vi "Configure Dialog.vi"(8 "error in (no error)":errorcluster, 11 "Create Channel Arbitrary Waveform [ACH] Msg in":refnum<class "Create Channel Arbitrary Waveform [ACH] Msg.lvclass">) -> (0 "error out":errorcluster, 2 "Ok?":bool, 3 "Create Channel Arbitrary Waveform [ACH] Msg out":refnum<class "Create Channel Arbitrary Waveform [ACH] Msg.lvclass">)   [LabVIEW 2014, in "CS++Fgen.lvlib" / "Create Channel Arbitrary Waveform [ACH] Msg.lvclass"]
uses:
  Create Channel Arbitrary Waveform [ACH] Msg.lvclass
  Create Channel Arbitrary Waveform [ACH] Msg.lvclass/Create Channel Arbitrary Waveform [ACH] Msg.ctl
panel:
  in  "Channel Name (\"\")":string="CHANNEL1" caption="Channel Name"
  in  "waveform data array (empty)":dbl[](array[numeric]) caption="Waveform Data Array"
  in  "OK Button":bool
  in  "Cancel Button":bool
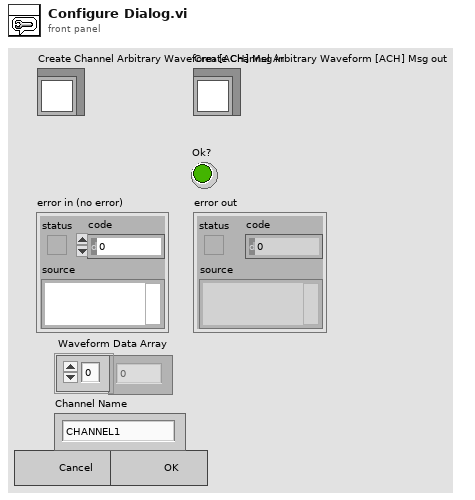
[diagram p1: front panel]
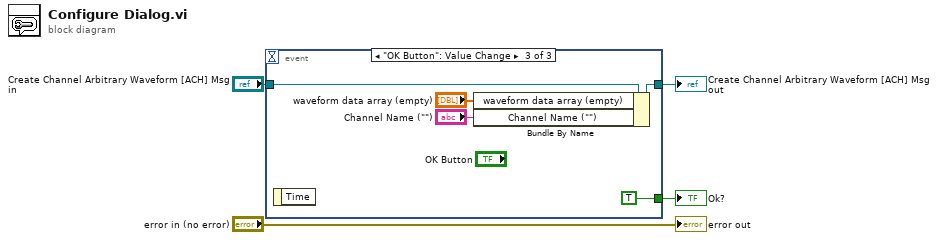
[diagram p0: block diagram]
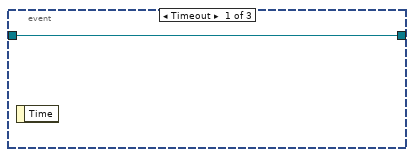
[diagram p2: hidden frame]
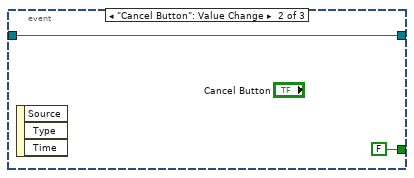
[diagram p3: hidden frame]
diagram:
  n1 = event shown="[2] \"OK Button\": Value Change" {
    selector: _ -> [_ _ _]
    dyn-events: _ -> [_ _ _]
    timeout: _ -> [_ _ _]
    tunnel: [w5 w7 w10] -> w3
    tunnel: "Create Channel Arbitrary Waveform [ACH] Msg in" -> [w5 w7 w12]
    tunnel: [_ FALSE TRUE] -> w1
    event Timeout {
      n2 = event-data() -> ()  [unwired: 1 in, 1 out]
    }
    event "Cancel Button": Value Change {
      n3 = event-data() -> ()  [unwired: 1 in, 3 out]
    }
    event "OK Button": Value Change {
      n4 = event-data() -> ()  [unwired: 1 in, 1 out]
      n5 = Bundle By Name(cluster=w12, "waveform data array (empty)"="waveform data array (empty)", "Channel Name (\"\")"="Channel Name (\"\")") -> (w10:refnum<class "Create Channel Arbitrary Waveform [ACH] Msg.lvclass">)
    }
  }
  "Create Channel Arbitrary Waveform [ACH] Msg out" <- w3
  "Ok?" <- w1
  "error out" <- "error in (no error)"
